vi "Reset Buffers.vi"(8 "error in (no error)":errorcluster, 11 "Top Level in":refnum<class "Top Level.lvclass">) -> (0 "error out":errorcluster, 3 "Top Level out":refnum<class "Top Level.lvclass">)   [LabVIEW 2021, in "Top Level.lvlib" / "Top Level.lvclass"]
uses:
  Top Level.lvclass
  Top Level.lvclass/Top Level.ctl
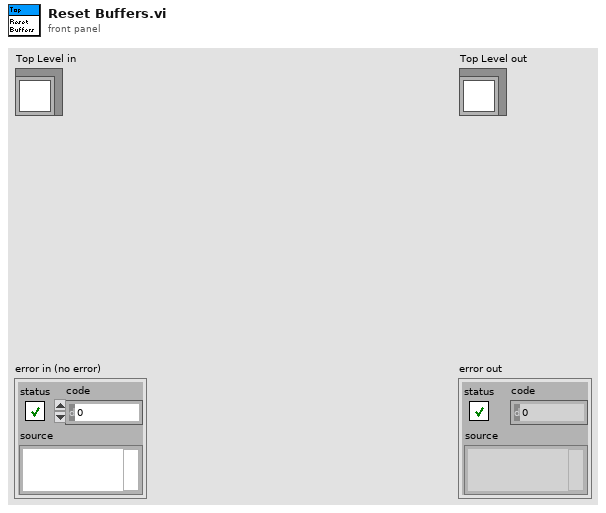
[diagram p1: front panel]
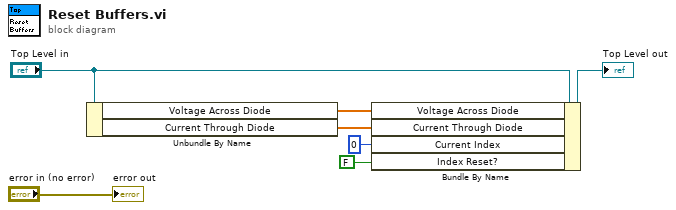
[diagram p0: block diagram]
diagram:
  n1 = Unbundle By Name("Top Level in") -> ("Voltage Across Diode"=w3:dbl[], "Current Through Diode"=w4:dbl[])
  n2 = Bundle By Name(cluster="Top Level in", "Voltage Across Diode"=w3, "Current Through Diode"=w4, "Current Index"=0 ("Acquisition.Current Index"), "Index Reset?"=FALSE) -> (→"Top Level out":refnum<class "Top Level.lvclass">)
  "error out" <- "error in (no error)"
